vi "HXSortTerm.vi"(1 "Terms":T19, 2 "State In":T1 {"BlockNodeState"."Draw Style" items=["FunctionBlock", "ExpressVI", "Variable", "Elemental I/O", "32x32 Icon", "FunctionBlockCompact"]; "BlockNodeState"."Terminal Data"."Terminal Flags" format="%.0b"}) -> (0 "Array":T21[](array[typedef]))   [LabVIEW 2017]
uses:
  <vilib>/XNodeSupport/XNodeTermRef.ctl
  <vilib>/XNodeSupport/XNodeTermIDPairs.ctl
  <vilib>/XNodeSupport/XNodeTermIDPair.ctl
  <vilib>/XNodeSupport/XNodeString.ctl
  <vilib>/Platform/storage/lvStorage.llb/xStorage/Write Data/State.ctl
  <vilib>/BlockNodeSupport/BlockNodeState.ctl
  <vilib>/BlockNodeSupport/TerminalData.ctl
  <vilib>/picture/picture.llb/imagedata.ctl
  <vilib>/Platform/storage/lvStorage.llb/dataStorageParams.ctl
  <vilib>/Platform/storage/lvStorage.llb/_selectedProp.ctl
  <vilib>/Platform/storage/lvStorage.llb/dataModel.ctl
  <vilib>/Platform/storage/Storage.llb/usiTypeDef.ctl
  <vilib>/Platform/storage/Storage.llb/usiPropDef.ctl
  <vilib>/express/express shared/ex_EditUserDefinedProperties/usiDataType.ctl
  <vilib>/Platform/storage/Storage.llb/specialProperties.ctl
  <vilib>/Platform/storage/Storage.llb/usiOverwriteOptions.ctl
  <vilib>/Platform/storage/lvStorage.llb/TerminalDef.ctl
  <vilib>/Platform/storage/lvStorage.llb/_TerminalStyle.ctl
  <vilib>/Utility/XNodeSupport.llb/XRect32.ctl
  <vilib>/Platform/storage/Storage.llb/usiSequenceRepresentation.ctl
  <vilib>/Platform/storage/lvStorage.llb/channelType.ctl
  <vilib>/Platform/storage/lvStorage.llb/_dataTerminals.ctl
  <vilib>/XNodeSupport/NI_XNodeSupport.lvlib
  <vilib>/Platform/storage/lvStorage.llb/xStorage/Write Data/Write Data.xnode
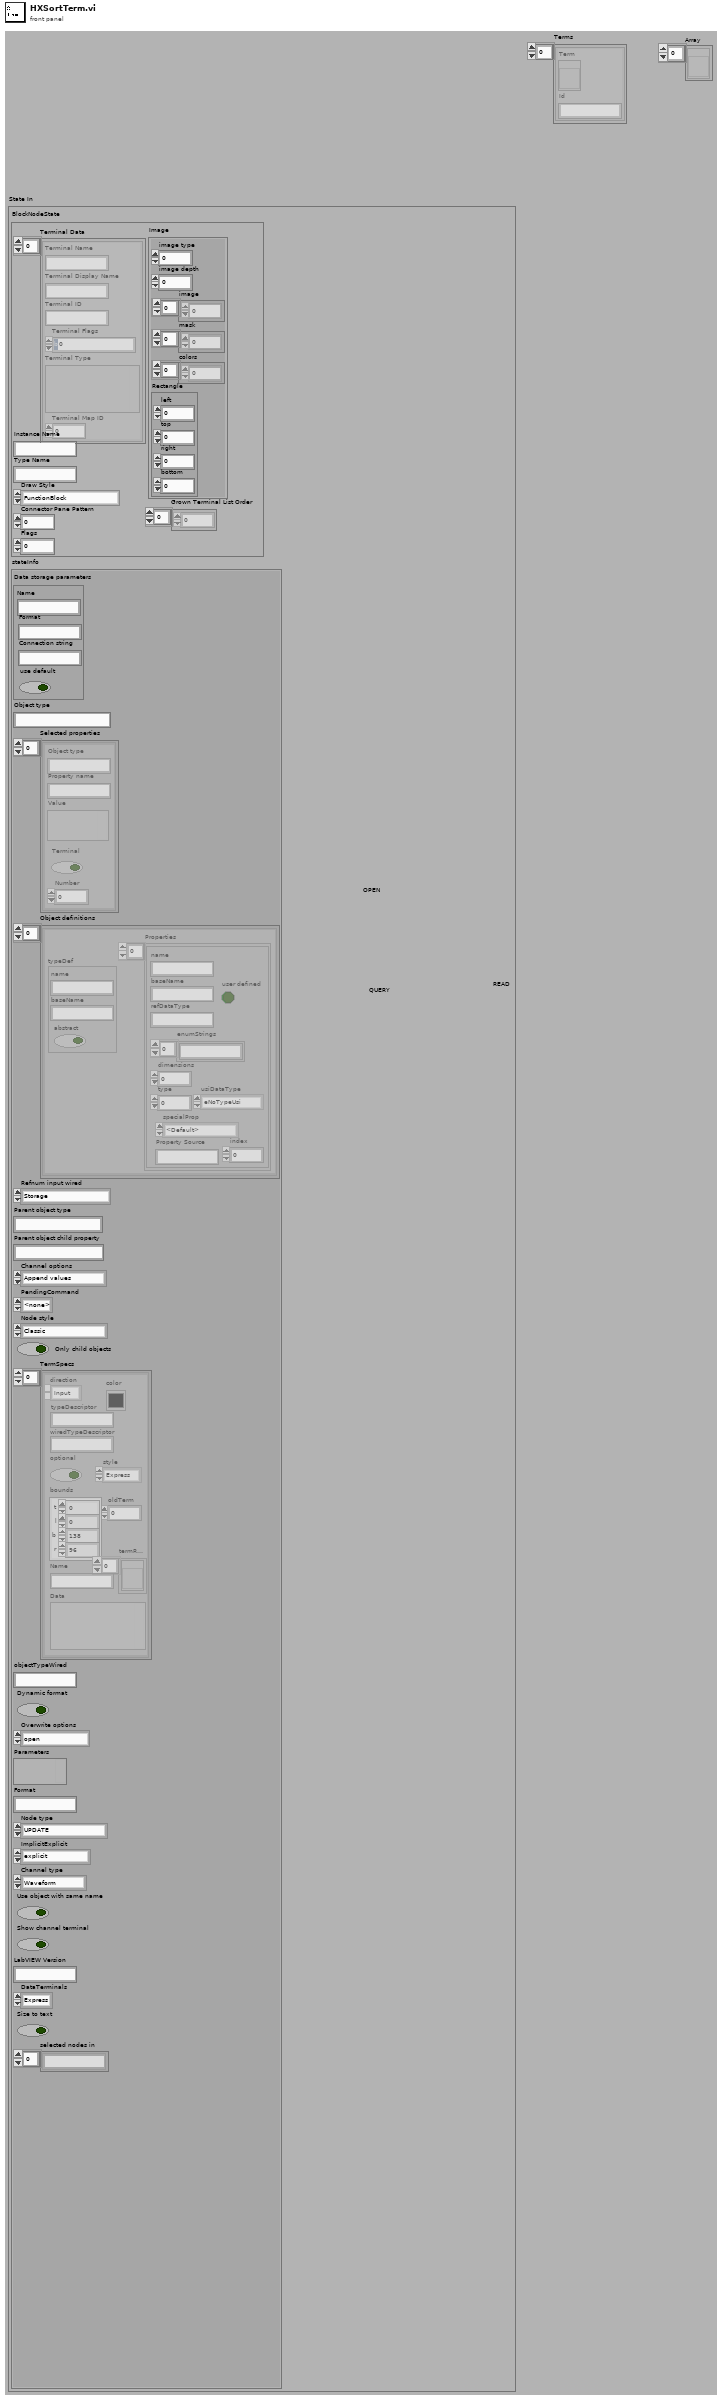
[diagram p1: front panel]
types:
  T1 = typedef "Write Data.xnode/State.ctl" = cluster{"BlockNodeState":T2, "stateInfo":cluster{"Data storage parameters":T5, "Object type":string, "Selected properties":T6[], "Object definitions":T7[], "Refnum input wired":enum16{"Storage", "Generic object", "Typed object", "<none>"}, "Parent object type":string, "Parent object child property":string, "Channel options":T12, "PendingCommand":enum16{"<none>", "SelPopUp", "Init"}, "Node style":enum16{"Classic", "Express"}, "Only child objects":bool, "TermSpecs":T13[], "objectTypeWired":string, "Dynamic format":bool, "Overwrite options":enum16{"open", "open or create", "create or replace", "create", "open (read only)"}, "Parameters":variant, "Format":string, "Node type":enum16{"UPDATE", "READ", "QUERY", "CREATE CHILD", "CREATE", "CONNECT", "DISCONNECT"}, "ImplicitExplicit":T16, "Channel type":T17, "Use object with same name":bool, "Show channel terminal":bool, "LabVIEW Version":string, "DataTerminals":T18, "Size to text":bool, "selected nodes in":string[]}}
  T2 = typedef "BlockNodeState.ctl" = cluster{"Terminal Data":T3[], "Instance Name":string, "Type Name":string, "Draw Style":i32, "Connector Pane Pattern":i32, "Flags":i32, "Grown Terminal List Order":i32[], "Image":T4}
  T3 = typedef "TerminalData.ctl" = cluster{"Terminal Name":string, "Terminal Display Name":string, "Terminal ID":string, "Terminal Flags":i32, "Terminal Type":variant, "Terminal Map ID":i32}
  T4 = typedef "imagedata.ctl" = cluster{"image type":i32, "image depth":i32, "image":u8[], "mask":u8[], "colors":u32[], "Rectangle":cluster{"left":i16, "top":i16, "right":i16, "bottom":i16}}
  T5 = typedef "dataStorageParams.ctl" = cluster{"Name":string, "Format":string, "Connection string":string, "use default":bool}
  T6 = typedef "_selectedProp.ctl" = cluster{"Object type":string, "Property name":string, "Value":variant, "Terminal":bool, "Number":i32}
  T7 = typedef "dataModel.ctl" = cluster{"typeDef":T8, "Properties":T9[]}
  T8 = typedef "usiTypeDef.ctl" = cluster{"name":string, "baseName":string, "abstract":bool}
  T9 = typedef "usiPropDef.ctl" = cluster{"name":string, "baseName":string, "refDataType":string, "dimensions":i32, "type":i32, "user defined":bool, "enumStrings":string[], "usiDataType":T10, "specialProp":T11, "Property Source":string, "index":i32}
  T10 = typedef "usiDataType.ctl" = enum16{"eNoTypeUsi", "eInt8Usi", "eInt16Usi", "eInt32Usi", "eInt64Usi", "eUInt8Usi", "eUInt16Usi", "eUInt32Usi", "eUInt64Usi", "eFloat32Usi", "eFloat64Usi", "- 0", "- 1", "- 2", "- 3", "- 4", "- 5", "- 6", "- 7", "- 8", "- 9", "eString8Usi", "eString16Usi", "eStringUsi", "eEnumUsi", "- 10", "- 11", "- 12", "- 13", "- 14", "eTimeUsi", "- 15", "- 16", "- 17", "- 18", "- 19", "- 20", "- 21", "- 22", "- 23", "eInstanceUsi", "eStoreUsi"}
  T11 = typedef "specialProperties.ctl" = enum16{"<Default>", "Channel Values", "AppendReplace", "ChannelFlags", "ValueFlags", "ImplicitExplicit", "InsertIndex", "ValuesCount", "ComparisonOperator", "Cluster", "DAQmx Channel"}
  T12 = typedef "usiOverwriteOptions.ctl" = enum16{"Append values", "Replace values at index", "Replace all values", "Append if timeline aligns"}
  T13 = typedef "TerminalDef.ctl" = cluster{"direction":enum16{"Input", "Output"}, "typeDescriptor":string, "color":u32, "oldTerm":i32, "style":T14, "optional":bool, "bounds":T15, "termRefs":refnum<vi>[], "Name":string, "Data":variant, "wiredTypeDescriptor":string}
  T14 = typedef "_TerminalStyle.ctl" = enum16{"Express", "Collapsed", "Internal"}
  T15 = typedef "XRect32.ctl" = cluster{"t":i32, "l":i32, "b":i32, "r":i32}
  T16 = typedef "usiSequenceRepresentation.ctl" = enum16{"explicit", "implicit"}
  T17 = typedef "channelType.ctl" = enum16{"Waveform", "Array of Double", "Array of String", "DDT", "Array of UInt8", "Array of Int16", "Array of Int32", "Array of Single", "Array of DateTime", "Array of Waveform", "none", "DateTime", "String", "Double", "Single", "UInt8", "Int16", "Int32"}
  T18 = typedef "_dataTerminals.ctl" = enum16{"Express", "Cluster"}
  T19 = typedef "NI_XNodeSupport.lvlib/XNodeTermIDPairs.ctl" = T20[]
  T20 = typedef "NI_XNodeSupport.lvlib/XNodeTermIDPair.ctl" = cluster{"Term":T21, "Id":T22}
  T21 = typedef "NI_XNodeSupport.lvlib/XNodeTermRef.ctl" = refnum<vi>
  T22 = typedef "NI_XNodeSupport.lvlib/XNodeString.ctl" = string
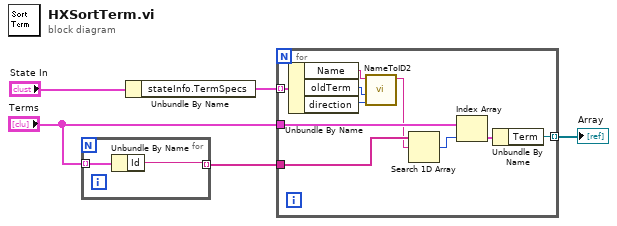
[diagram p0: block diagram]
diagram:
  n1 = for {
    tunnel: "Terms" -> [w7] mode=indexing
    tunnel: [w6] -> w4 mode=indexing
    n2 = Unbundle By Name(w7) -> ("Id"=w6:T22)
  }
  n3 = Unbundle By Name("State In") -> ("stateInfo.TermSpecs"=w3:T13[])
  n4 = for {
    tunnel: w3 -> [w12] mode=indexing
    tunnel: w4 -> [w17]
    tunnel: "Terms" -> [w16]
    tunnel: [w13] -> w1 mode=indexing
    n5 = Unbundle By Name(w12) -> ("Name"=w11:string, "oldTerm"=w10:i32, "direction"=w9:enum16{"Input", "Output"})
    n6 = call <vilib>:"NameToID2.vi"("direction"=w9, "old term"=w10, "name"=w11) -> ("String Out"=w8:string)  [unwired: 8 in]
    n7 = Search 1D Array(1D array=w17, element=w8) -> (index of element=w15:i32)  [unwired: 1 in]
    n8 = Index Array(array=w16, index=w15) -> (element=w14:T20)
    n9 = Unbundle By Name(w14) -> ("Term"=w13:T21)
  }
  "Array" <- w1
